vi "Copy Golden Template to User Location.vi"(8 "Error In":errorcluster, 9 "Bus Number":i32, 10 "Destination Path":path=path "C:/Users/kvemishe/Downloads", 11 "Golden Template Source Path":path=path "C:/Users/kvemishe/Desktop/Test") -> (0 "error out":errorcluster, 3 "Curent Bus Path":path)   [LabVIEW 2014]
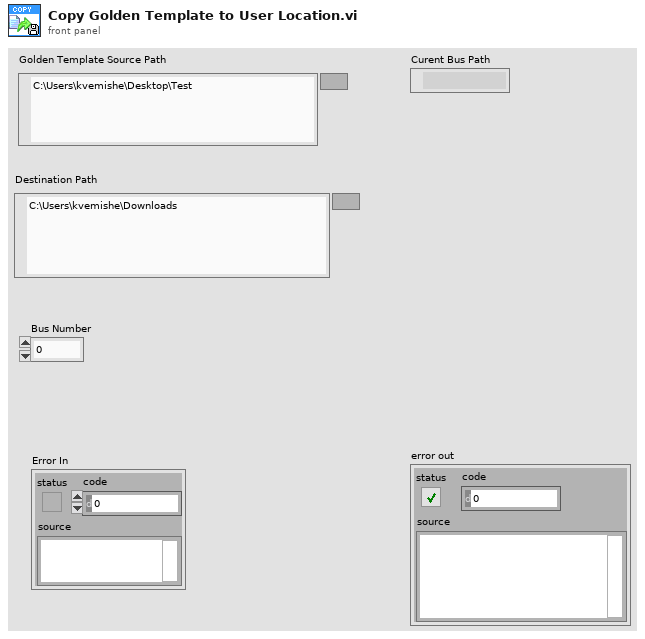
[diagram p1: front panel]
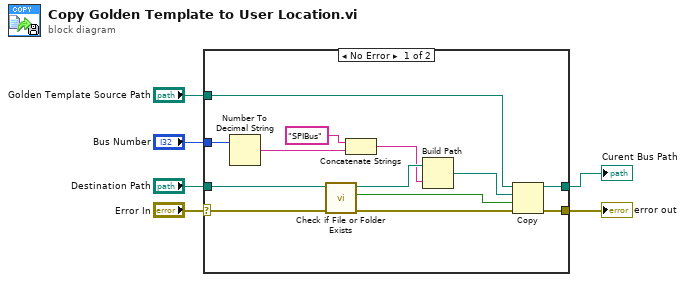
[diagram p0: block diagram]
diagram:
  n1 = case shown="No Error" "Error In" {
    selector: "Error In" -> [w18 w20]
    tunnel: "Golden Template Source Path" -> [w19 w21]
    tunnel: [w16 w20] -> w4
    tunnel: "Destination Path" -> [w14 _]
    tunnel: "Bus Number" -> [w11 _]
    tunnel: [w7 w21] -> w1
    frame No Error {
      n2 = Number To Decimal String(number=w11) -> (decimal integer string=w9:string)  [unwired: 1 in]
      n3 = call <vilib>:"Check if File or Folder Exists.vi"("error in (no error)"=w18, "path"=w14) -> ("error out"=w17:errorcluster, "file or folder exists?"=w15:bool, "dup path"=w13:path)  [unwired: 7 in]
      n4 = Concatenate Strings("SPIBus" ("string"), w9) -> (w8:string)
      n5 = Build Path(base path=w13, name or relative path=w8) -> (appended path=w12:path)
      n6 = Copy(8:w17, 9:w15, 10:w12, 11:w19) -> (0:w16:errorcluster, 3:w7:path)  [unwired: 1 in, 1 out]
    }
    frame Error {
    }
  }
  "error out" <- w4
  "Curent Bus Path" <- w1
